vi "舒张压报警.vi"(1 "舒张压下限":dbl, 2 "舒张压上限":dbl, 3 "舒张压":dbl, 4 "警示 2":refnum<vi>) -> (0 "预警 2":string)   [LabVIEW 2016]
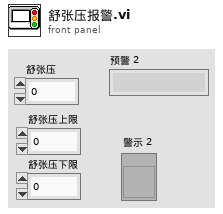
[diagram p1: front panel]
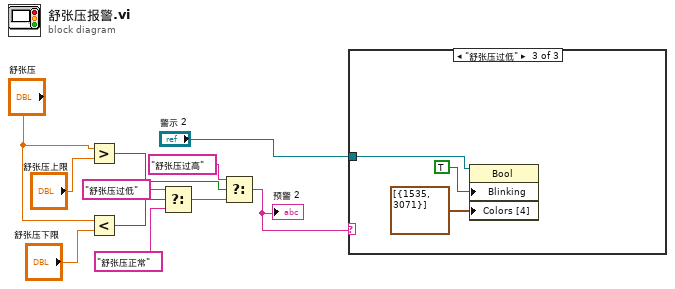
[diagram p0: block diagram]
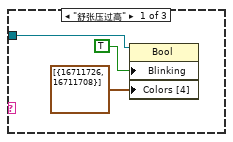
[diagram p2: hidden frame]
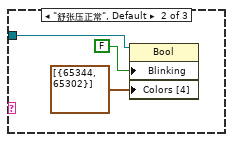
[diagram p3: hidden frame]
diagram:
  n1 = Greater?(x="舒张压", y="舒张压上限") -> (0:w10:bool)
  n2 = Less?(x="舒张压", y="舒张压下限") -> (x < y?=w7:bool)
  n3 = Select(t="舒张压过低", s=w7, f="舒张压正常") -> (s? t:f=w9:string)
  n4 = Select(t="舒张压过高", s=w10, f=w9) -> (s? t:f=w3:string)
  "预警 2" <- w3
  n5 = case shown="\"舒张压过低\"" w3 {
    tunnel: "警示 2" -> [w14 w15 w18]
    frame "舒张压过高" {
      n6 = property class="Bool"(reference=w14, "Blinking"=TRUE ("闪烁"), "Colors [4]"=cluster{u32, u32}[] [{16711726, 16711708}] ("颜色[4]")) -> ()  [unwired: 1 in, 2 out]
    }
    frame "舒张压正常", Default {
      n7 = property class="Bool"(reference=w15, "Blinking"=FALSE ("闪烁"), "Colors [4]"=cluster{u32, u32}[] [{65344, 65302}] ("颜色[4]")) -> ()  [unwired: 1 in, 2 out]
    }
    frame "舒张压过低" {
      n8 = property class="Bool"(reference=w18, "Blinking"=TRUE ("闪烁"), "Colors [4]"=cluster{u32, u32}[] [{1535, 3071}] ("颜色[4]")) -> ()  [unwired: 1 in, 2 out]
    }
  }
